vi "PostCopyScripting.vi"(10 "MetaDataObj":refnum<class "MetaDataObj.lvclass">, 11 "User Project":refnum<vi>) -> ()   [LabVIEW 2013, in "DCAFConfigurablePluginDecideFeatures.lvclass"]
uses:
  DCAFConfigurablePluginDecideFeatures.lvclass
  <resource>/dialog/NewProjectWizard/MetaDataObj/MetaDataObj.lvclass
  DCAFConfigurablePluginDecideFeatures.lvclass/DCAFConfigurablePluginDecideFeatures.ctl
  Read component name.vi
  <vilib>/Utility/EditLVLibs/Edit LVLibs.lvlib
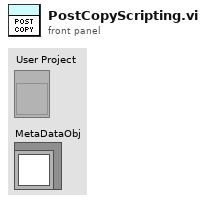
[diagram p1: front panel]
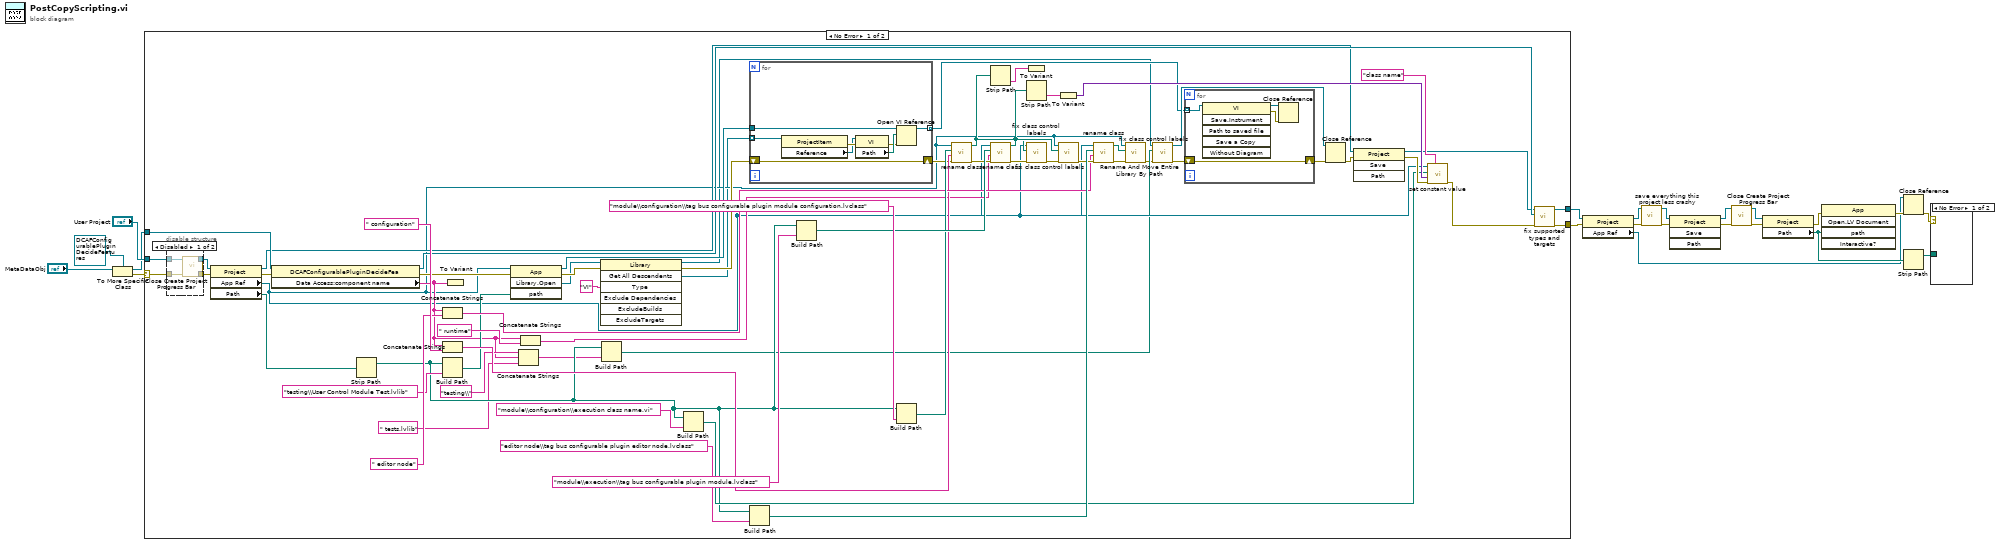
[diagram p0: block diagram]
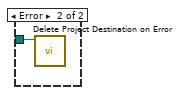
[diagram p2: hidden frame]
diagram:
  n1 = To More Specific Class(target class=refnum<class "DCAFConfigurablePluginDecideFeatures.lvclass"> refnum ("DecideProjectFeatures.lvclass"), reference="MetaDataObj") -> (specific class reference=w14:refnum<class "DCAFConfigurablePluginDecideFeatures.lvclass">, error out=w19:errorcluster)  [unwired: 1 in]
  n2 = case shown="No Error" w19 {
    selector: w19 -> [w67 w104]
    tunnel: [w55 w105] -> w11
    tunnel: "User Project" -> [w66 w105]
    tunnel: [w56 w104] -> w10
    tunnel: w14 -> [w81 _]
    frame No Error {
      n3 = disable-structure shown="Disabled" {
        disable-tunnel: w67 -> [w89 w90]
        disable-tunnel: w66 -> [w88 w91]
        disable-tunnel: [w87 w91] -> w65
        disable-tunnel: [w86 w90] -> w64
        frame Disabled {
          n4 = call <resource>:"Close Create Project Progress Bar.vi"("error in (no error)"=w89, "Project"=w88) -> ("error out"=w86:errorcluster, "dup Project"=w87:refnum<vi>)  [unwired: 8 in]
        }
        frame Enabled {
        }
      }
      n5 = property class="Project"(reference=w65, error in=w64) -> (reference out=w71:refnum<vi>, error out=w85:errorcluster, "App Ref"=w31:refnum<vi>, "Path"=w84:path)
      n6 = property class="DCAFConfigurablePluginDecideFea"(reference=w81, error in=w85) -> (reference out=w76:refnum<class "DCAFConfigurablePluginDecideFeatures.lvclass">, error out=w39:errorcluster, "Data Access:component name"=w32:string)
      n7 = Strip Path(path=w84) -> (stripped path=w36:path)  [unwired: 1 out]
      n8 = Concatenate Strings(w32, " editor node" ("string")) -> (w57:string)
      n9 = Concatenate Strings(w32, " configuration" ("string")) -> (w53:string)
      n10 = Build Path(base path=w36, name or relative path="testing\\User Control Module Test.lvlib") -> (appended path=w37:path)
      n11 = To Variant(anything=w32) -> ()  [unwired: 1 out]
      n12 = invoke class="App" method="Library.Open"(reference=w31, error in=w39, "path"=w37) -> (reference out=w41:refnum<vi>, error out=w45:errorcluster, "Open Library"=w44:refnum<vi>)  [unwired: 1 in, 1 out]
      n13 = Concatenate Strings("testing\\" ("string"), w32, " tests.lvlib" ("string")) -> (w34:string)
      n14 = Concatenate Strings(w32, " runtime" ("string")) -> (w46:string)
      n15 = invoke class="Library" method="Get All Descendents"(reference=w44, error in=w45, "Type"="VI") -> (reference out=w24:refnum<vi>, error out=w42:errorcluster, "All Descendents"=w25:refnum<vi>[])  [unwired: 4 in, 4 out]
      n16 = Build Path(base path=w36, name or relative path=w34) -> (appended path=w23:path)
      n17 = Build Path(base path=w36, name or relative path="module\\configuration\\execution class name.vi") -> (appended path=w52:path)
      n18 = for {
        tunnel: [w99] -> w27 mode=indexing
        shift-right: [w98] -> w40
        shift-left: w42 -> [w98]
        tunnel: w41 -> [w97]
        tunnel: w25 -> [w96] mode=indexing
        n19 = property class="ProjectItem"(reference=w96) -> (error out=w103:errorcluster, "Reference"=w102:refnum<vi>)  [unwired: 1 in, 1 out]
        n20 = property class="VI"(reference=w102, error in=w103) -> (error out=w100:errorcluster, "Path"=w101:path)  [unwired: 1 out]
        n21 = Open VI Reference(application reference (local)=w97, vi path=w101, error in (no error)=w100) -> (vi reference=w99:refnum<vi>)  [unwired: 3 in, 1 out]
      }
      n22 = Build Path(base path=w36, name or relative path="editor node\\tag bus configurable plugin editor node.lvclass") -> (appended path=w62:path)
      n23 = Build Path(base path=w36, name or relative path="module\\execution\\tag bus configurable plugin module.lvclass") -> (appended path=w80:path)
      n24 = Build Path(base path=w36, name or relative path="module\\configuration\\tag bus configurable plugin module configuration.lvclass") -> (appended path=w77:path)
      n25 = call "rename class.vi"("error in"=w40, "new name"=w53, "class path"=w77, "Application in"=w31) -> ("error out"=w78:errorcluster, "New Library Path"=w48:path)  [unwired: 6 in]
      n26 = Strip Path(path=w48) -> (name=w49:string)  [unwired: 1 out]
      n27 = call "rename class.vi"("error in"=w78, "new name"=w46, "class path"=w80, "Application in"=w31) -> ("error out"=w69:errorcluster, "New Library Path"=w50:path)  [unwired: 6 in]
      n28 = To Variant(anything=w49) -> ()  [unwired: 1 out]
      n29 = Strip Path(path=w50) -> (name=w51:string)  [unwired: 1 out]
      n30 = call "fix class control labels.vi"("error in"=w69, "class to load"=w48, "Application in"=w31) -> ("error out"=w68:errorcluster)  [unwired: 8 in]
      n31 = To Variant(anything=w51) -> (Variant=w75:variant)
      n32 = call "fix class control labels.vi"("error in"=w68, "class to load"=w50, "Application in"=w31) -> ("error out"=w59:errorcluster)  [unwired: 8 in]
      n33 = call "rename class.vi"("error in"=w59, "new name"=w57, "class path"=w62, "Application in"=w31) -> ("error out"=w60:errorcluster, "New Library Path"=w61:path)  [unwired: 6 in]
      n34 = call "fix class control labels.vi"("error in"=w60, "class to load"=w61, "Application in"=w31) -> ("error out"=w22:errorcluster)  [unwired: 8 in]
      n35 = call <vilib>:"Rename And Move Entire Library By Path.vi"("error in (no error)"=w22, "New library path"=w23, "Library ref in"=w24) -> ("error out"=w29:errorcluster, "Library ref out"=w30:refnum<vi>)  [unwired: 7 in]
      n36 = for {
        tunnel: w27 -> [w95] mode=indexing
        shift-right: [w92] -> w28
        shift-left: w29 -> [w92]
        n37 = invoke class="VI" method="Save.Instrument"(reference=w95) -> (reference out=w93:refnum<vi>, error out=w94:errorcluster)  [unwired: 5 in, 4 out]
        n38 = Close Reference(reference=w93, error in (no error)=w94) -> ()  [unwired: 1 out]
      }
      n39 = Close Reference(reference=w30, error in (no error)=w28) -> (error out=w26:errorcluster)
      n40 = invoke class="Project" method="Save"(reference=w71, error in=w26) -> (reference out=w70:refnum<vi>, error out=w72:errorcluster)  [unwired: 2 in, 2 out]
      n41 = call "set constant value.vi"("control name"="class name", "error in"=w72, "data to set"=w75, "vi path"=w52, "Application in"=w31) -> ("error out"=w54:errorcluster)  [unwired: 6 in]
      n42 = call "fix supported types and targets.vi"("error in"=w54, "DecideProjectFeatures in"=w76, "User Project in"=w70) -> ("error out"=w56:errorcluster, "User Project out"=w55:refnum<vi>)  [unwired: 7 in]
    }
    frame Error {
    }
  }
  n43 = property class="Project"(reference=w11, error in=w10) -> (reference out=w8:refnum<vi>, error out=w9:errorcluster, "App Ref"=w7:refnum<vi>)
  n44 = call "save everything this project less crashy.vi"("error in"=w9, "Project in"=w8) -> ("error out"=w13:errorcluster, "Project out"=w12:refnum<vi>)  [unwired: 8 in]
  n45 = invoke class="Project" method="Save"(reference=w12, error in=w13) -> (reference out=w3:refnum<vi>, error out=w4:errorcluster)  [unwired: 2 in, 2 out]
  n46 = call <resource>:"Close Create Project Progress Bar.vi"("error in (no error)"=w4, "Project"=w3) -> ("error out"=w1:errorcluster, "dup Project"=w2:refnum<vi>)  [unwired: 8 in]
  n47 = property class="Project"(reference=w2, error in=w1) -> (error out=w18:errorcluster, "Path"=w15:path)  [unwired: 1 out]
  n48 = invoke class="App" method="Open.LV Document"(error in=w18, "path"=w15) -> (error out=w17:errorcluster)  [unwired: 3 in, 4 out]
  n49 = Close Reference(reference=w7, error in (no error)=w17) -> (error out=w6:errorcluster)
  n50 = Strip Path(path=w15) -> (stripped path=w5:path)  [unwired: 1 out]
  n51 = case shown="No Error" w6 {
    tunnel: w5 -> [_ w106]
    frame No Error {
    }
    frame Error {
      n52 = call <resource>:"Delete Project Destination on Error.vi"("Project Destination Root"=w106) -> ()  [unwired: 11 in]
    }
  }
